vi "DSF.Shared.Configuration.Plugin.Get Timing.vi"(11 "Plugin Configuration in":refnum<class "DSF.Shared.Configuration.Plugin.lvclass">) -> (2 "Timing":refnum<class "DSF.Engine.Timing.lvclass">, 3 "Plugin Configuration out":refnum<class "DSF.Shared.Configuration.Plugin.lvclass">)   [LabVIEW 2016, in "DSF.Shared.lvlib" / "DSF.Shared.Configuration.Plugin.lvclass"]
uses:
  DSF.Shared.Configuration.Plugin.lvclass
  Engine/Classes/Timing/DSF.Engine.Timing.lvclass
  DSF.Shared.Configuration.Plugin.lvclass/DSF.Shared.Configuration.Plugin.ctl
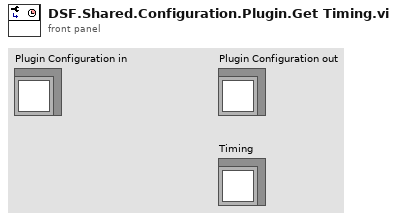
[diagram p1: front panel]
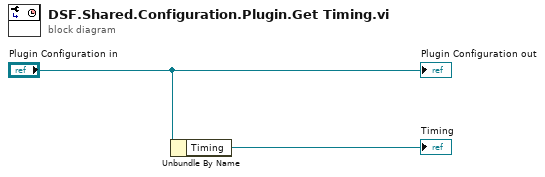
[diagram p0: block diagram]
diagram:
  n1 = Unbundle By Name("Plugin Configuration in") -> ("Timing"=→"Timing":refnum<class "DSF.Engine.Timing.lvclass">)
  "Plugin Configuration out" <- "Plugin Configuration in"
